vi "RichToFlatniswitch_grpc_SelfTestResponse.vi"(5 "OutputClusterType":T1, 11 "InputCluster":T2) -> (3 "OutputCluster":T1)   [LabVIEW 2021, in "NI Switch_client.lvlib"]
uses:
  NI Switch_client.lvlib
  niswitch_grpc_SelfTestResponse_Flat.ctl
  niswitch_grpc_SelfTestResponse.ctl
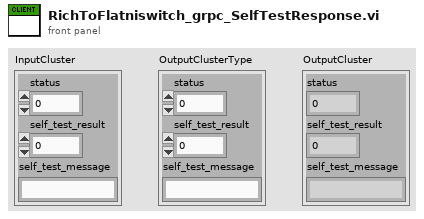
[diagram p1: front panel]
types:
  T1 = typedef "NI Switch_client.lvlib/niswitch_grpc_SelfTestResponse_Flat.ctl" = cluster{"status":i32, "self_test_result":i32, "self_test_message":string}
  T2 = typedef "NI Switch_client.lvlib/niswitch_grpc_SelfTestResponse.ctl" = cluster{"status":i32, "self_test_result":i32, "self_test_message":string}
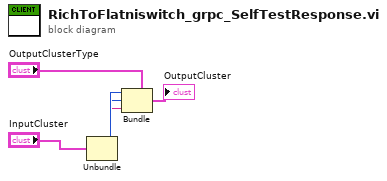
[diagram p0: block diagram]
diagram:
  n1 = Unbundle "Unbundle"("InputCluster") -> ("status"=w3:i32, "self_test_result"=w2:i32, "self_test_message"=w1:string)
  n2 = Bundle "Bundle"(cluster="OutputClusterType", "status"=w3, "self_test_result"=w2, "self_test_message"=w1) -> (→"OutputCluster":T1)
